vi "Get BLISS_Poll Server (SubVI).vi"(8 "error in":errorcluster, 11 "Data Parameters in":T1={"Start Time"=timestamp(3690155740.033191 s since 1904-01-01), "Save to Folder"=path "", "Forces in Theater"=[{"Force Commander"="BlissUT124", "Units"=[]}, {"Force Commander"="BlissMP146", "Units"=[]}, {"Force Commander"="BlissMP145", "Units"=[]}, {"Force Commander"="BlissMP140", "Units"=[]}, {"Force Commander"="BlissMP137", "Units"=[]}, {"Force Commander"="BlissMP135", "Units"=[]}, {"Force Commander"="BlissMP134", "Units"=[]}, {"Force Commander"="BlissMP132", "Units"=[]}, {"Force Commander"="BlissMA109", "Units"=[]}, {"Force Commander"="BlissMA107", "Units"=[]}, {"Force Commander"="BlissMA106", "Units"=[]}, {"Force Commander"="BlissMA101", "Units"=[]}, {"Force Commander"="BlissLU118", "Units"=[]}, {"Force Commander"="BlissLU117", "Units"=[]}, {"Force Commander"="BlissLU116", "Units"=[]}, {"Force Commander"="BlissLU115", "Units"=[]}, {"Force Commander"="BlissLU114", "Units"=[]}, {"Force Commander"="BlissLU113", "Units"=[]}, {"Force Commander"="BlissLU111", "Units"=[]}, {"Force Commander"="BlissLL185", "Units"=[]}, {"Force Commander"="BlissLL183", "Units"=[]}, {"Force Commander"="BlissLL173", "Units"=[]}, {"Force Commander"="BlissLL172", "Units"=[]}, {"Force Commander"="BlissLL171", "Units"=[]}, {"Force Commander"="BlissJH103", "Units"=[]}, {"Force Commander"="BlissJH102", "Units"=[]}, {"Force Commander"="BlissJH101", "Units"=[]}, {"Force Commander"="BlissJE116", "Units"=[]}, {"Force Commander"="BlissJE115", "Units"=[]}, {"Force Commander"="BlissJE114", "Units"=[]}, {"Force Commander"="BlissJE111", "Units"=[]}, {"Force Commander"="BlissHD183", "Units"=[]}, {"Force Commander"="BlissHD182", "Units"=[]}, {"Force Commander"="BlissHD181", "Units"=[]}, {"Force Commander"="BlissGPDFFPL", "Units"=[]}, {"Force Commander"="BlissEUWIPES", "Units"=[]}, {"Force Commander"="BlissEU179", "Units"=[]}, {"Force Commander"="BlissEU178", "Units"=[]}, {"Force Commander"="BlissEU177", "Units"=[]}, {"Force Commander"="Blissdvds02", "Units"=[]}, {"Force Commander"="BlissDOWIPES", "Units"=[]}, {"Force Commander"="BlissCR022", "Units"=[]}, {"Force Commander"="BlissCR021", "Units"=[]}, {"Force Commander"="BlissCG167", "Units"=[]}, {"Force Commander"="BlissCG166", "Units"=[]}, {"Force Commander"="BlissCG161", "Units"=[]}, {"Force Commander"="BlissCG160", "Units"=[]}, {"Force Commander"="BlissCG159", "Units"=[]}, {"Force Commander"="BlissCG158", "Units"=[]}, {"Force Commander"="BlissCG157", "Units"=[]}, {"Force Commander"="BlissCG156", "Units"=[]}, {"Force Commander"="BlissCG151", "Units"=[]}, {"Force Commander"="BlissCB172", "Units"=[]}, {"Force Commander"="BlissCB171", "Units"=[]}, {"Force Commander"="BlissCB108", "Units"=[]}, {"Force Commander"="BlissCB107", "Units"=[]}, {"Force Commander"="BlissBV181", "Units"=[]}, {"Force Commander"="BlissBV162", "Units"=[]}, {"Force Commander"="BlissAK177", "Units"=[]}, {"Force Commander"="BlissAK176", "Units"=[]}, {"Force Commander"="BlissAK175", "Units"=[]}, {"Force Commander"="BlissAK174", "Units"=[]}, {"Force Commander"="BlissAK173", "Units"=[]}, {"Force Commander"="BlissAK172", "Units"=[]}, {"Force Commander"="BlissAK171", "Units"=[]}, {"Force Commander"="BlissAK139", "Units"=[]}, {"Force Commander"="BlissAK134", "Units"=[]}, {"Force Commander"="BlissAK131", "Units"=[]}, {"Force Commander"="BlissAH163", "Units"=[]}, {"Force Commander"="BlissAH162", "Units"=[]}, {"Force Commander"="BlissAH161", "Units"=[]}, {"Force Commander"="BlissAH122", "Units"=[]}, {"Force Commander"="BlissAH121", "Units"=[]}, {"Force Commander"="BlissAD106", "Units"=[]}, {"Force Commander"="BlissAD104", "Units"=[]}, {"Force Commander"="BlissAB105", "Units"=[]}, {"Force Commander"="BlissAB104", "Units"=[]}]}) -> (0 "error out":errorcluster, 3 "Data Parameters out":T1, 5 "Aborting Process":bool)   [LabVIEW 2020]
uses:
  MC5e Gobal_Variables.vi
  MC5e Squad_Info.ctl
  MC5e Unit_Status_List.ctl
  MC5e Data_Parameters.ctl
  MC5e Terrain types.ctl
  Location.ctl
  MC5e Unit.ctl
  MC5e Force.ctl
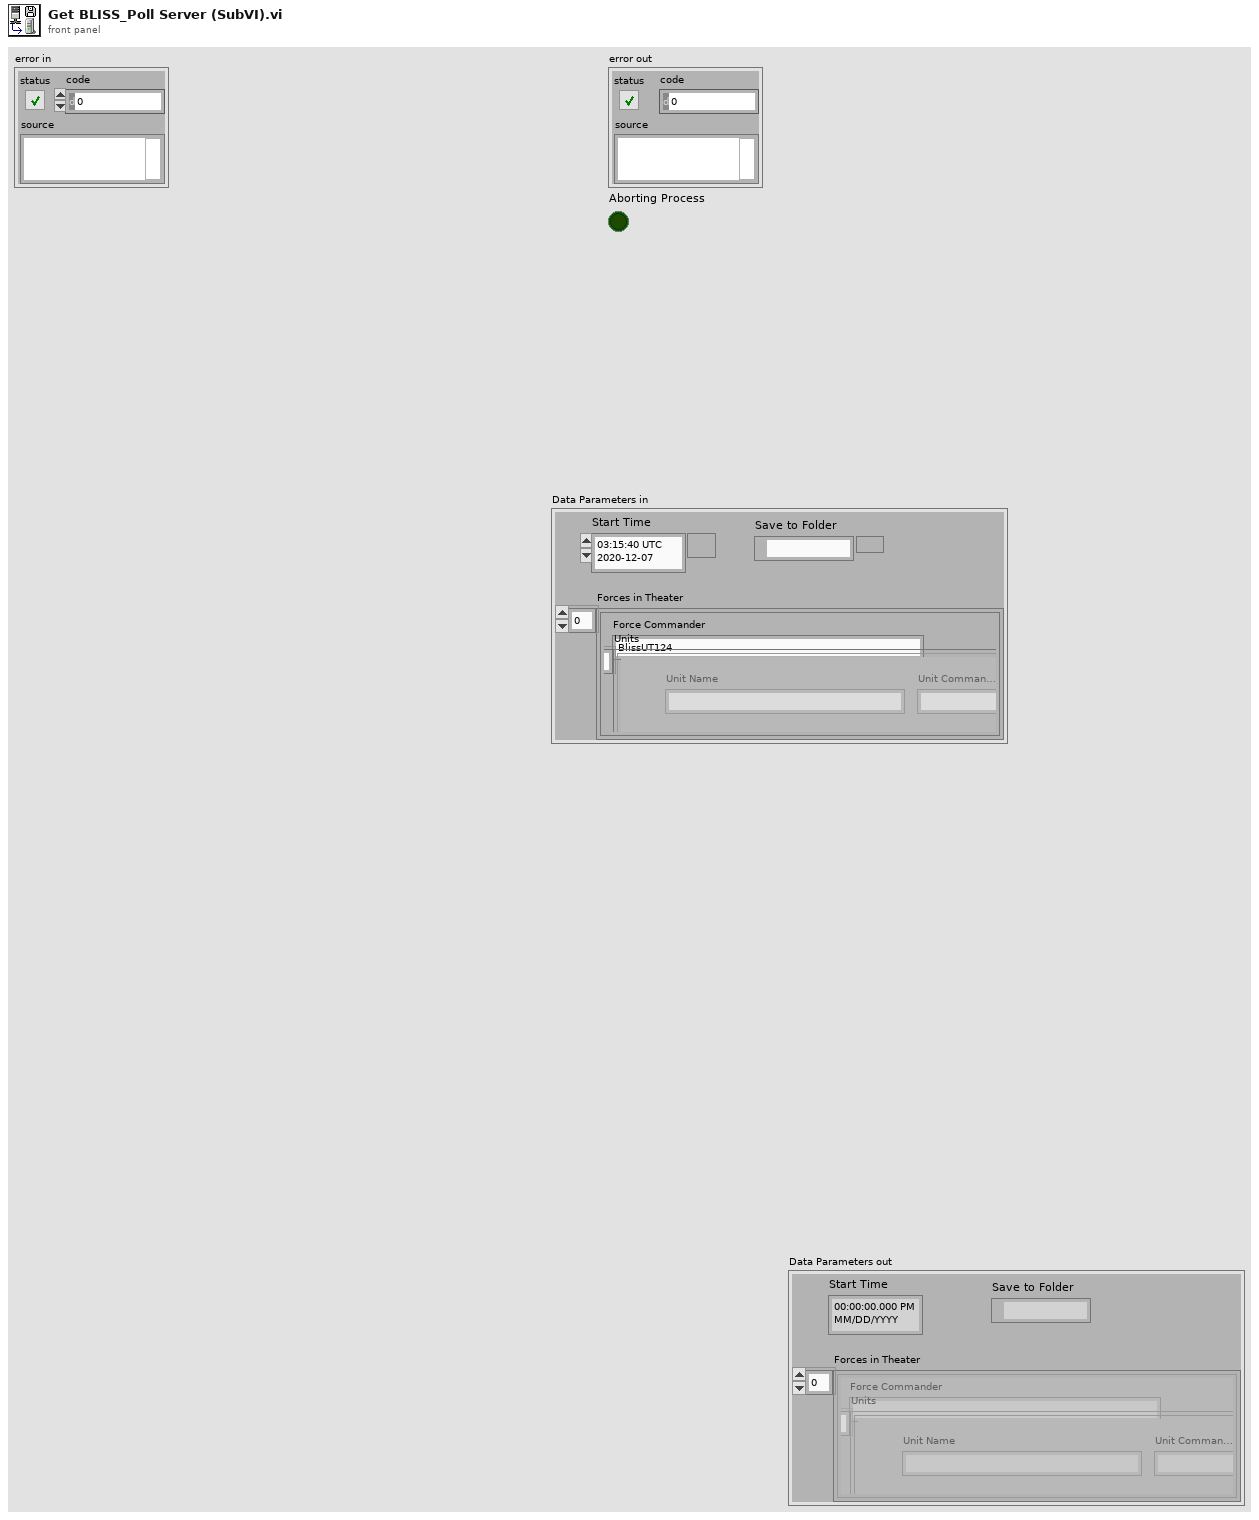
[diagram p1: front panel]
types:
  T1 = typedef "MC5e Data_Parameters.ctl" = cluster{"Start Time":timestamp, "Save to Folder":path, "Forces in Theater":T2[]}
  T2 = typedef "MC5e Force.ctl" = cluster{"Force Commander":string, "Units":T3[]}
  T3 = typedef "MC5e Unit.ctl" = cluster{"Squad List":T4, "Unit Fatigue Level":enum16{"Not Fatigued", "Fatigued", "Seriously Fatigued"}, "Flying Unit":bool, "Mounted Unit":bool, "Difficult Terrain Types":T6, "Full BR":dbl, "Defending from Stronghold":bool, "Speed":dbl, "Capacity %":dbl, "Morale":dbl, "Current BR":dbl, "Location":T7, "Unit Name":string, "Unit Commander":string, "Unit Notes":string}
  T4 = typedef "MC5e Unit_Status_List.ctl" = T5[]
  T5 = typedef "MC5e Squad_Info.ctl" = cluster{"Squad Name":string, "# Soldiers":dbl, "Battle Rating":dbl, "Flying":bool, "Mounted":bool, "Speed":dbl, "Range":dbl, "Morale":dbl, "Token Image":variant, "Max Endurance":dbl, "Current Endurance":dbl, "Difficult Terrain":T6}
  T6 = typedef "MC5e Terrain types.ctl" = cluster{"Artic / snow / ice)":bool, "Coast":bool, "Desert / sand":bool, "Forest / woodland":bool, "Grassland / plains":bool, "Mountain / canyons":bool, "Underdark / caverns":bool, "Acquatic / rivers, lakes, ocean":bool}
  T7 = typedef "Location.ctl" = cluster{"X coordinate":dbl, "Y coordinate":dbl}
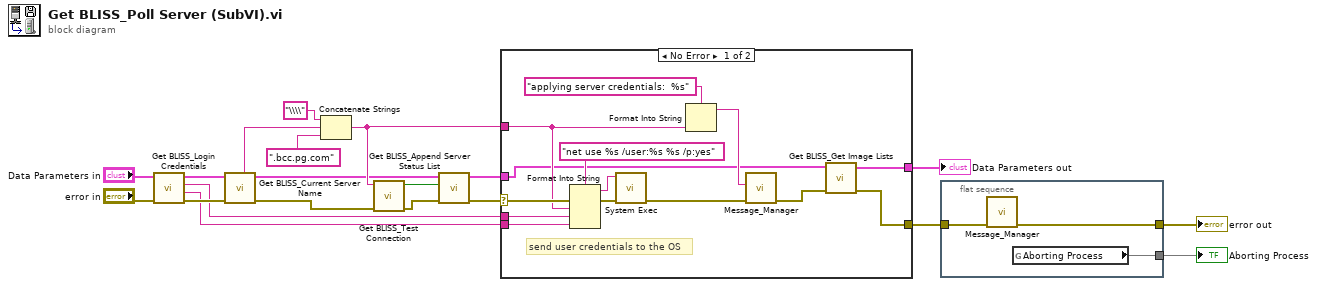
[diagram p0: block diagram]
diagram:
  n1 = call "Get BLISS_Login Credentials.vi"("error in"="error in", "Data Parameters in"="Data Parameters in") -> ("error out"=w13:errorcluster, "password"=w11:string, "username (e.g. name.i@pg.com)"=w12:string, "Data Parameters out"=w2:T1)  [unwired: 6 in]
  n2 = call "Get BLISS_Current Server Name.vi"("error in"=w13, "Data Parameters in"=w2) -> ("error out"=w15:errorcluster, "Data Parameters out"=w6:T1, "Server Name"=w7:string)  [unwired: 6 in, 1 out]
  n3 = Concatenate Strings("\\\\" ("string"), w7, ".bcc.pg.com" ("string")) -> (w10:string)
  n4 = call "Get BLISS_Test Connection.vi"("error in (no error)"=w15, "server"=w10) -> ("error out"=w9:errorcluster, "Valid"=w1:bool)  [unwired: 8 in]
  n5 = call "Get BLISS_Append Server Status List.vi"("error in"=w9, "Valid Connection"=w1, "Data Parameters in"=w6) -> ("error out"=w8:errorcluster, "Data Parameters out"=w5:T1)  [unwired: 7 in]
  n6 = case shown="No Error" w8 {
    selector: w8 -> [w31 w36]
    tunnel: [w30 w36] -> w18
    tunnel: w10 -> [w24 _]
    tunnel: w12 -> [w29 _]
    tunnel: w11 -> [w28 _]
    tunnel: w5 -> [w23 w35]
    tunnel: [w22 w35] -> w4
    frame No Error {
      # "send user credentials to the OS"
      n7 = Format Into String(format string="net use %s /user:%s %s /p:yes", error in=w31, w24, w29, w28) -> (resulting string=w32:string, error out=w33:errorcluster)  [unwired: 1 in]
      n8 = call <vilib>:"System Exec.vi"("error in (no error)"=w33, "command line"=w32) -> ("error out"=w21:errorcluster)  [unwired: 6 in, 3 out]
      n9 = Format Into String(format string="applying server credentials:  %s" ("New Entry"), w24) -> (resulting string=w27:string)  [unwired: 2 in, 1 out]
      n10 = call "Message_Manager.vi"("error in"=w21, "New Entry"=w27) -> ("error out"=w25:errorcluster)  [unwired: 4 in, 5 out]
      n11 = call "Get BLISS_Get Image Lists.vi"("error in"=w25, "Data Parameters in"=w23) -> ("error out"=w30:errorcluster, "Data Parameters out"=w22:T1)  [unwired: 8 in]
    }
    frame Error {
    }
  }
  "Data Parameters out" <- w4
  n12 = flat-sequence {
    tunnel: [w37] -> w16
    tunnel: w18 -> [w38]
    tunnel: [w39] -> w17
    frame #0 {
      n13 = call "Message_Manager.vi"("error in"=w38) -> ("error out"=w37:errorcluster)  [unwired: 5 in, 5 out]
      n14 = global read "MC5e Gobal_Variables.vi" "Aborting Process"() -> (w39)
    }
  }
  "error out" <- w16
  "Aborting Process" <- w17
